vi "Typecast Queue to Refnum.vi"(11 "queue in":T1) -> (3 "refnum out":T2)   [LabVIEW 2010, in "NI_LVConfig.lvlib"]
uses:
  NI_LVConfig.lvlib
  Config Data RefNum.ctl
  Config Queue.ctl
  Config Data.ctl
  Section.ctl
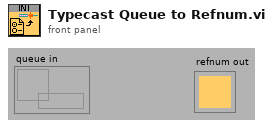
[diagram p1: front panel]
types:
  T1 = typedef "NI_LVConfig.lvlib/Config Queue.ctl" = refnum<queue>
  T2 = typedef "NI_LVConfig.lvlib/Config Data RefNum.ctl" = refnum<k1>
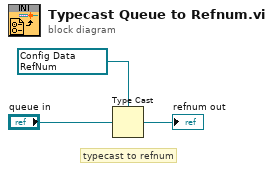
[diagram p0: block diagram]
diagram:
  w2 = T2 refnum items=["config data"] ("refnum out")
  # "typecast to refnum"
  n1 = Type Cast(type=w2, x="queue in") -> (*(type *) &x=→"refnum out":T2)
